vi "LaserParameter.vi"() -> ()   [LabVIEW 2011]
panel:
  in  "LaserParameter":string[](array[string])
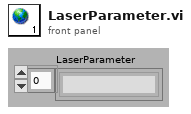
[diagram p1: front panel]
diagram:
